vi "IOPanel_4.vi"(11 "IOCard In":refnum<class "IOCard.lvclass">) -> ()   [LabVIEW 2019]
uses:
  Ctrl/IO Card_Type.ctl
  IO_Class/IOCard.lvclass
  <vilib>/Utility/miscctls.llb/LVPositionTypeDef.ctl
  IO_Class/IOCard.lvclass/IOCard.ctl
  LLB/Message/Ctrl/MsgDataInput.ctl
  LLB/Message/Ctrl/MsgPageSelect.ctl
  LLB/Message/Ctrl/LogType.ctl
  IO_Class/6480/6480.lvclass
  C:/Users/MyUser/Desktop/204J1_20201007/System/Function/IO Folder/IO_Class/IOCard.lvclass
  IO_Class/2410C/2410C-64.lvclass
  IO_Class/Zan/ZanCard.lvclass
  IO_Class/DMC1000B/DMC1000B.lvclass
  IO_Class/16InOut/16InOut.lvclass
  global/InAndOutGB.vi
  LLB/Commonly VI/Main Glb.vi
  <vilib>/Utility/config.llb/Read Key (String).vi
  LLB/Commonly VI.lvlib
  <vilib>/Utility/config.llb/NI_LVConfig.lvlib
  LLB/Message/MsgShowAndLog.lvlib
panel:
  out "IOCard":refnum<class "IOCard.lvclass">
  out "Card_Type":T1
  out "QName":string
  in  "Tab Control":enum32{"Input", "Output"}(tab)
  out "Lst_Input":i32[](listbox) caption="Input"
  in  "Lst_Output":i32[](listbox)=[2] caption="Output"
  out "CardNumber":i32
  out "IOType":enum16{"Input", "Output"}(ring)=enum."Output"
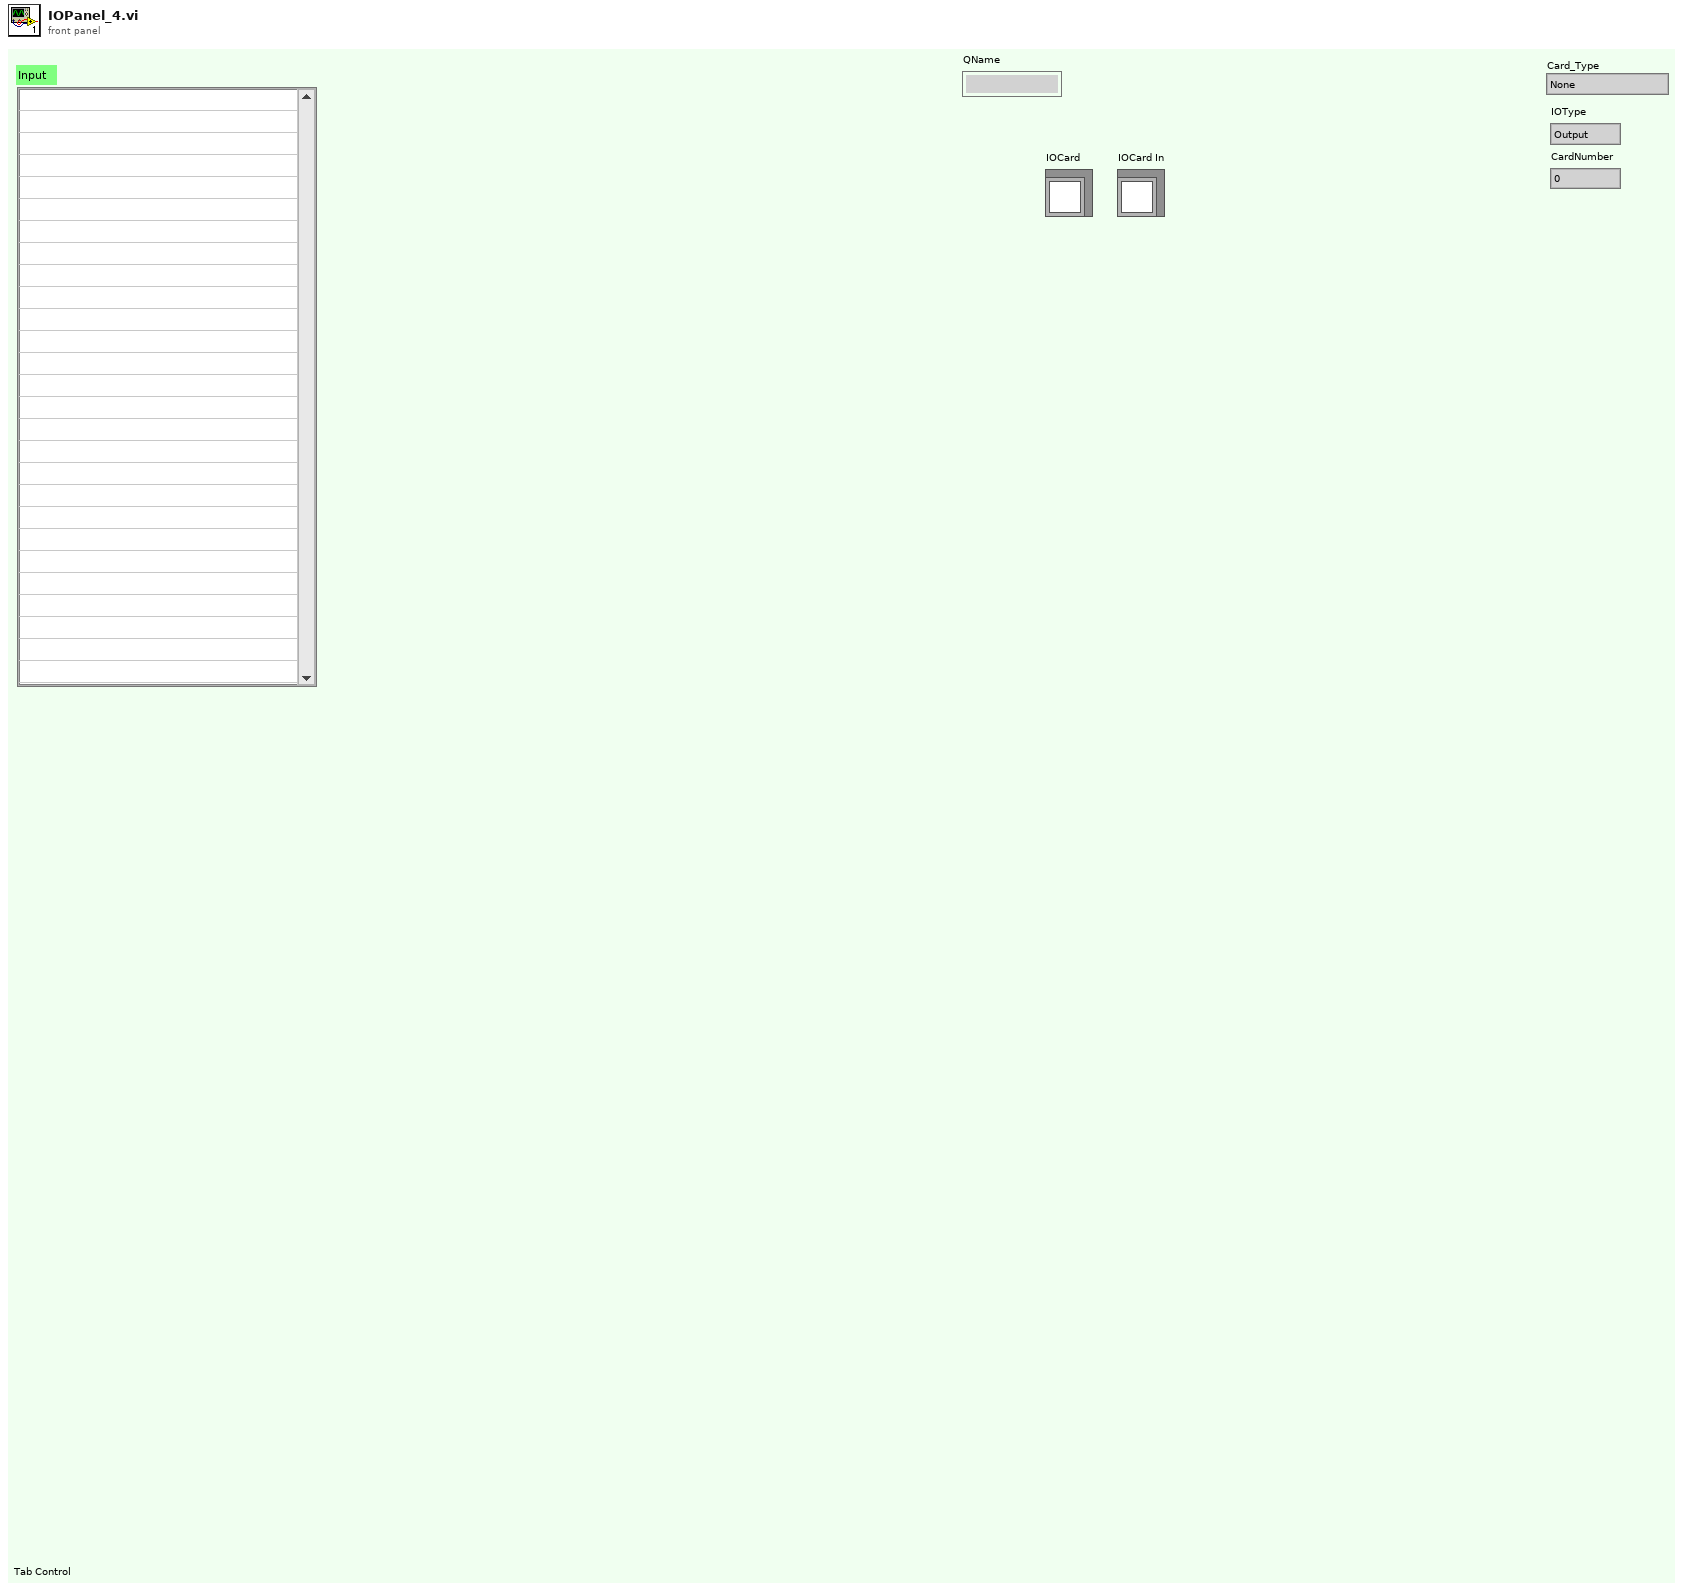
[diagram p1: front panel]
types:
  T1 = typedef "IO Card_Type.ctl" = enum16{"None", "Unidaq32", "6480", "2410C-64", "Zan", "DMC1000B", "16InOut", "Robot", "DMC3600"}
  T2 = typedef "LVPositionTypeDef.ctl" = cluster{"Left":i32, "Top":i32}
  T3 = cluster{"IO Card Type":T1, "IOType":enum16{"Input", "Output"}, "CardNumber":i32, "ConnectAct":bool, "IP":string}
  T4 = cluster{"CardNumber":i32, "Connect":bool, "Handler":i32}
  T5 = typedef "MsgDataInput.ctl" = cluster{"MsgPageSelect":T6, "LogType":T7, "Msg":string, "Time":string}
  T6 = typedef "MsgShowAndLog.lvlib/MsgPageSelect.ctl" = enum16{"System", "Comm", "IO", "Action", "Alarm"}
  T7 = typedef "MsgShowAndLog.lvlib/LogType.ctl" = enum16{"Auto", "Manual", "Handshake", "Error"}
  T8 = typedef "LVBoundsTypeDef.ctl" = cluster{"Width":u32, "Height":u32}
  T9 = typedef "LVPoint32TypeDef.ctl" = cluster{"Horizontal":i32, "Vertical":i32}
  T10 = typedef "NI_LVConfig.lvlib/Config Data RefNum.ctl" = refnum<k1>
  T11 = cluster{"Card":i32, "Connect":bool, "Handler":i32}[]
  T12 = cluster{"Card":i32, "Connect":bool, "Handler":i32}
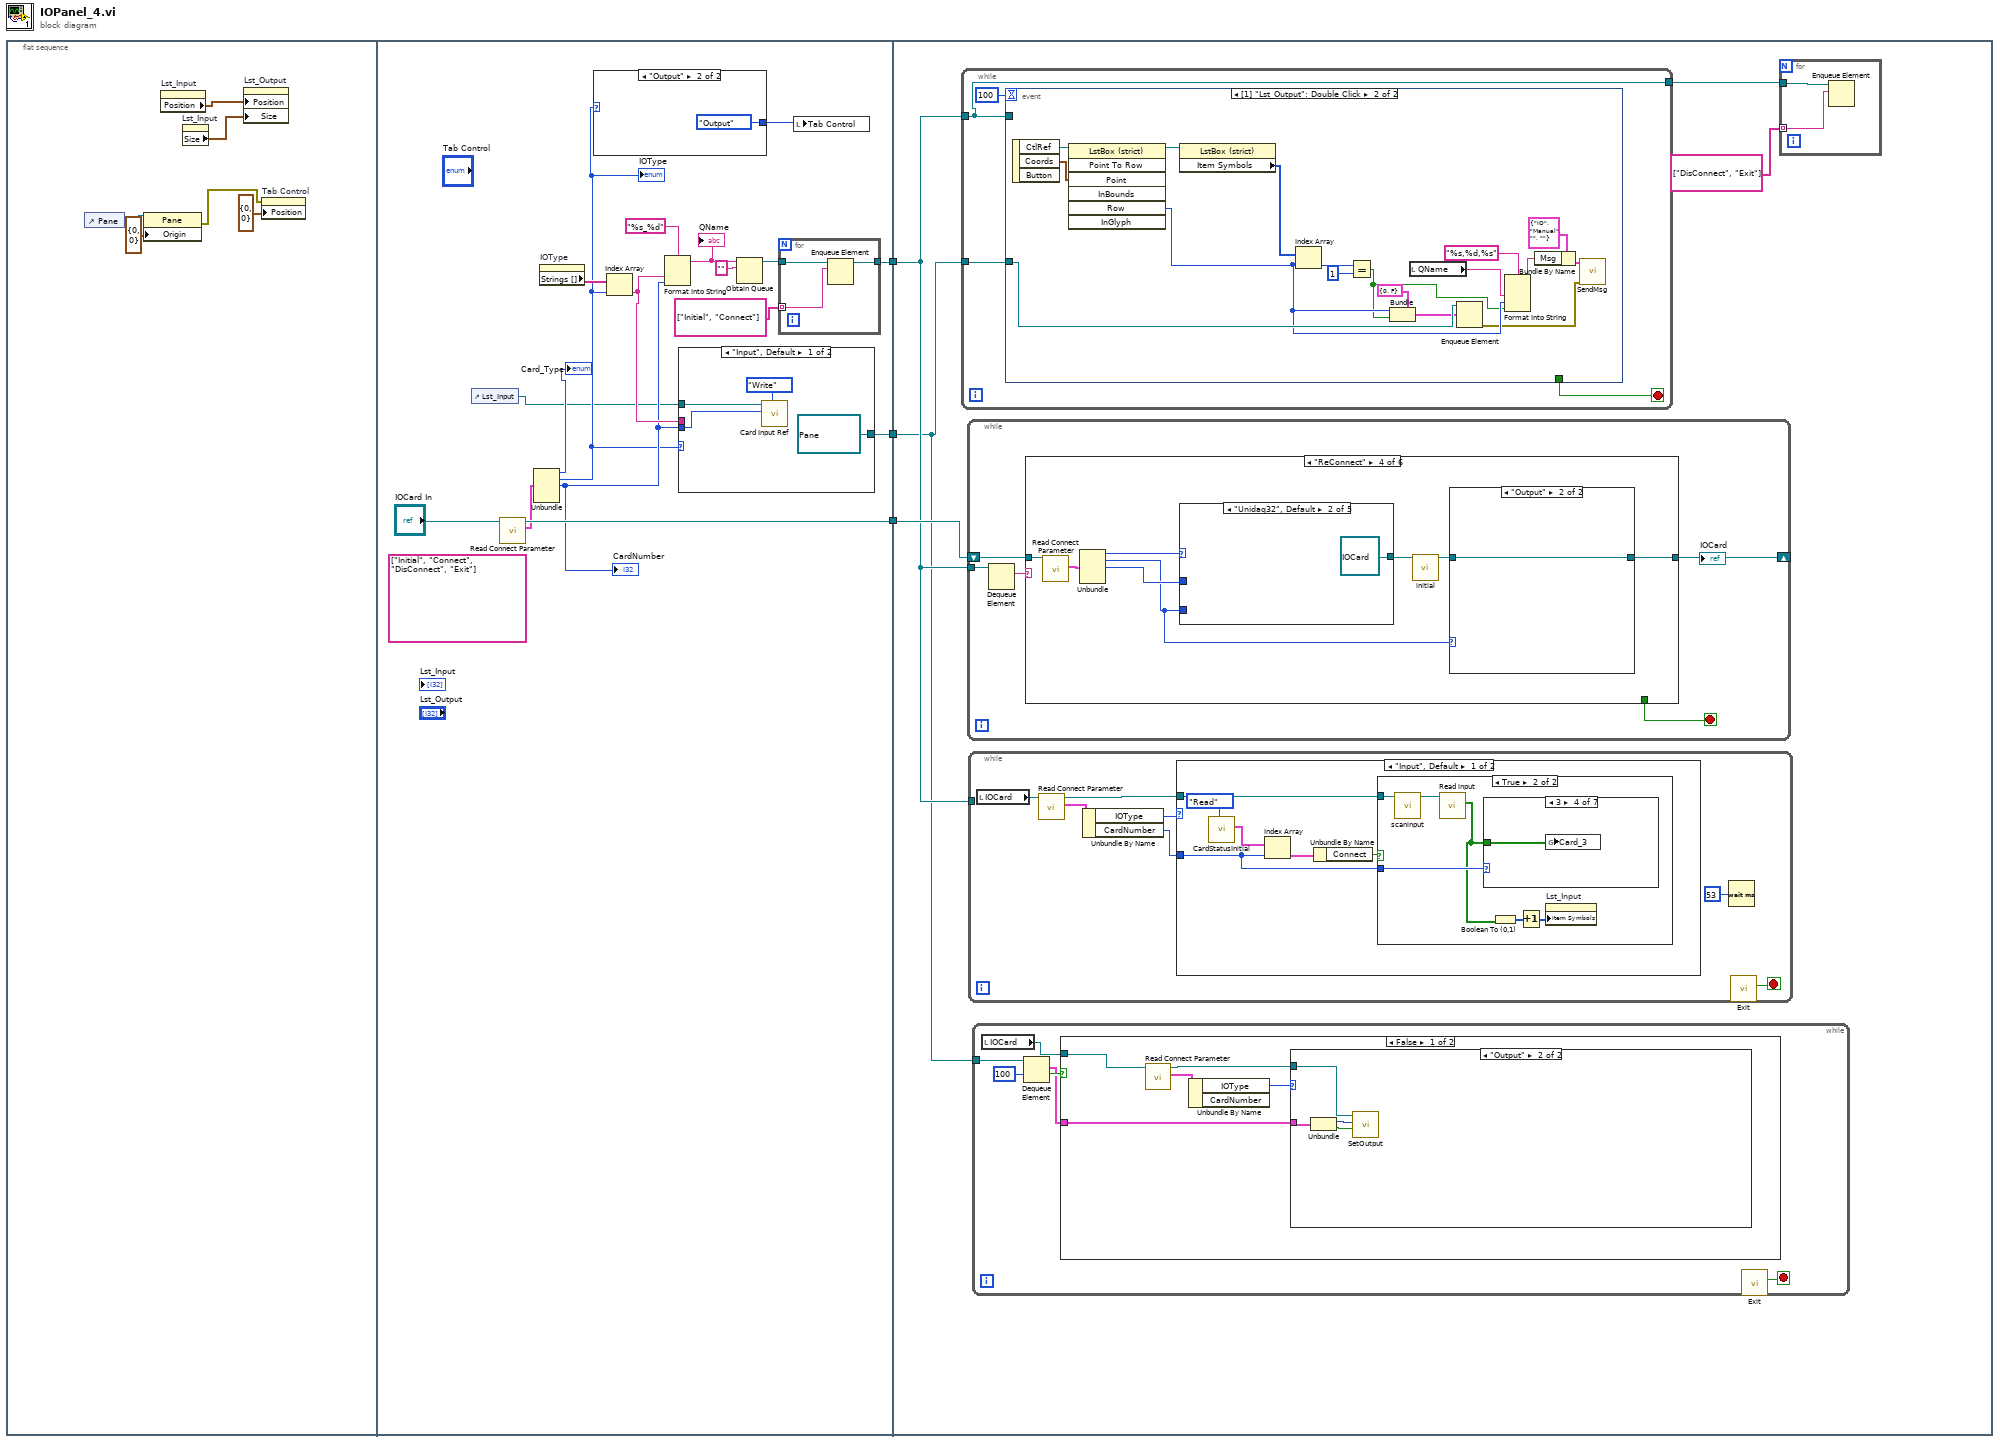
[diagram p0: block diagram]
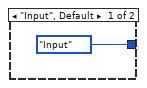
[diagram p2: hidden frame]
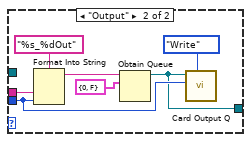
[diagram p3: hidden frame]
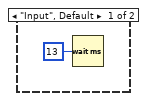
[diagram p4: hidden frame]
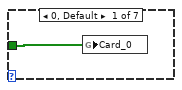
[diagram p7: hidden frame]
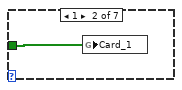
[diagram p8: hidden frame]
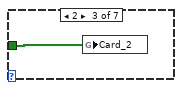
[diagram p9: hidden frame]
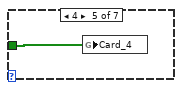
[diagram p10: hidden frame]
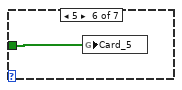
[diagram p11: hidden frame]
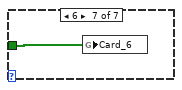
[diagram p12: hidden frame]
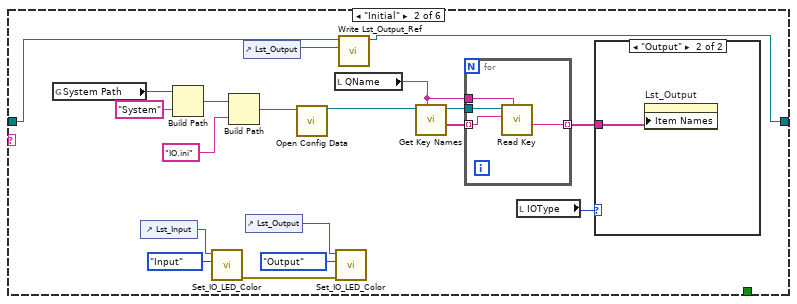
[diagram p15: hidden frame]
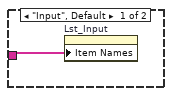
[diagram p16: hidden frame]
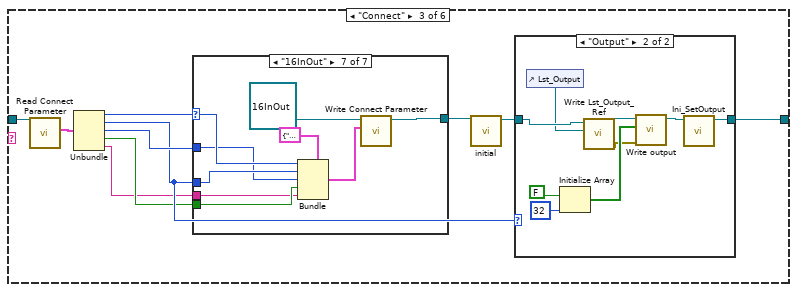
[diagram p17: hidden frame]
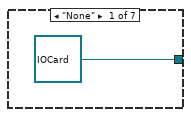
[diagram p19: hidden frame]
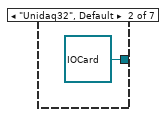
[diagram p20: hidden frame]
diagram:
  n1 = flat-sequence {
    tunnel: [w23] -> w3
    tunnel: [w18] -> w2
    tunnel: [w16] -> w1
    tunnel: w3 -> [w47]
    tunnel: w2 -> [w44]
    tunnel: w1 -> [w43]
    frame #0 {
      n2 = control-ref of="Pane"() -> (w6:refnum<vi>)
      n3 = property class="Pane"(reference=w6, "Origin"=T2 {"Left"=0, "Top"=0} ("Position")) -> (error out=w4:errorcluster)  [unwired: 1 in, 1 out]
      n4 = property on="Lst_Input" class="LstBox (strict)"() -> ("Position"=w8:T2)  [unwired: 2 in, 2 out]
      n5 = property on="Lst_Input" class="LstBox (strict)"() -> ("Size"=w9:T8)  [unwired: 2 in, 2 out]
      n6 = property on="Lst_Output" class="LstBox (strict)"("Position"=w8, "Size"=w9) -> ()  [unwired: 2 in, 2 out]
      n7 = property on="Tab Control" class="TabCtl (strict)"(error in=w4, "Position"=T2 {"Left"=0, "Top"=0}) -> ()  [unwired: 1 in, 2 out]
    }
    frame #1 {
      (unwired) string[] ["Initial", "Connect", "DisConnect", "Exit"]
      n8 = control-ref of="Lst_Input"() -> (w10:refnum<vi>)
      n9 = call "Read Connect Parameter.vi"("IOCard in"="IOCard In") -> ("Connect Parameter"=w22:T3, "IOCard out"=w23:refnum<class "IOCard.lvclass">)  [unwired: 8 in, 1 out]
      n10 = Unbundle(w22) -> ("IO Card Type"=→"Card_Type":T1, "IOType"=w12:enum16{"Input", "Output"}, "CardNumber"=w14:i32)  [unwired: 2 out]
      "CardNumber" <- w14
      "IOType" <- w12
      n11 = property on="IOType" class="Enum (strict)"() -> ("Strings []"=w21:string[])  [unwired: 2 in, 2 out]
      n12 = case shown="\"Output\"" w12 {
        tunnel: [enum32{"Input", "Output"}."Input" ("Tab Control") enum32{"Input", "Output"}."Output" ("Tab Control")] -> w11
        frame "Input", Default {
        }
        frame "Output" {
        }
      }
      n13 = Index Array(array=w21, index=w12) -> (element=w17:string)
      n14 = Format Into String(format string="%s_%d", w17, w14) -> (resulting string=w25:string)  [unwired: 2 in, 1 out]
      "QName" <- w25
      n15 = case shown="\"Input\", Default" w12 {
        tunnel: w17 -> [_ w37]
        tunnel: w14 -> [w29 w34]
        tunnel: [refnum<queue> refnum ("queue out") w33] -> w16
        tunnel: w10 -> [w30 _]
        frame "Input", Default {
          n16 = call "Card Input Ref.vi"("Action"=enum16{"Initial", "Write", "Read", "Release"}."Write", "CardIndex"=w29, "RefIn"=w30) -> ()  [unwired: 7 in, 2 out]
        }
        frame "Output" {
          n17 = Format Into String(format string="%s_%dOut", w37, w34) -> (resulting string=w39:string)  [unwired: 2 in, 1 out]
          n18 = Obtain Queue(name (unnamed)=w39, element data type=cluster{"Index":i32, "BL":bool} {"Index"=0, "BL"=FALSE}) -> (queue out=w33:refnum<queue>)  [unwired: 3 in, 2 out]
          n19 = call "Card Output Q.vi"("Action"=enum16{"Initial", "Write", "Read", "Release"}."Write", "CardIndex"=w34, "OutputQIn"=w33) -> ()  [unwired: 7 in, 2 out]
        }
      }
      n20 = Obtain Queue(name (unnamed)=w25, element data type="") -> (queue out=w19:refnum<queue>)  [unwired: 3 in, 2 out]
      n21 = for {
        tunnel: w19 -> [w42]
        tunnel: string[] ["Initial", "Connect"] -> [w41] mode=indexing
        tunnel: [w40] -> w18
        n22 = Enqueue Element(queue=w42, element=w41) -> (queue out=w40:refnum<queue>)  [unwired: 2 in, 2 out]
      }
      n23 = local write "Tab Control"(w11) -> ()
    }
    frame #2 {
      n24 = while {
        tunnel: w44 -> [w194]
        tunnel: [w194] -> w46
        tunnel: w43 -> [w193]
        stop <- w195 stop-if-true
        n25 = event shown="[1] \"Lst_Output\": Double Click" {
          selector: _ -> [_ _]
          dyn-events: _ -> [_ _]
          timeout: 100 -> [_ _]
          tunnel: [w197 _] -> w195
          tunnel: w194 -> [_ _]
          tunnel: w193 -> [_ w208]
          event Timeout {
            n26 = event-data() -> ()  [unwired: 1 in, 3 out]
            n27 = call "Exit.vi"() -> ("ExitOut"=w197:bool)  [unwired: 11 in]
          }
          event "Lst_Output": Double Click {
            n28 = event-data() -> ("CtlRef"=w214:refnum<vi>, "Coords"=w213:T9)  [unwired: 1 in, 1 out]
            n29 = invoke on="Invoke Node" class="LstBox (strict)" method="Point To Row"(reference=w214, "Point"=w213) -> (reference out=w209:refnum<vi>, "Row"=w200:i32)  [unwired: 5 in, 5 out]
            n30 = property on="Property Node" class="LstBox (strict)"(reference=w209) -> ("Item Symbols"=w212:i32[])  [unwired: 1 in, 2 out]
            n31 = Index Array(array=w212, index=w200) -> (element=w211:i32)
            n32 = Equal?(x=w211, y=1) -> (x = y?=w199:bool)
            n33 = Bundle(cluster=cluster{"Index":i32, "BL":bool} {"Index"=0, "BL"=FALSE} ("element"), "Index"=w200, "BL"=w199) -> (w207:cluster{"Index":i32, "BL":bool})
            n34 = local read "QName"() -> (w201:string)
            n35 = Enqueue Element(queue=w208, element=w207) -> (error out=w198:errorcluster)  [unwired: 2 in, 2 out]
            n36 = Format Into String(format string="%s,%d,%s", w201, w200, w199) -> (resulting string=w203:string)  [unwired: 2 in, 1 out]
            n37 = Bundle By Name(cluster=T5 {"MsgPageSelect"=enum."IO", "LogType"=enum."Manual", "Msg"="", "Time"=""} ("DataIn"), "Msg"=w203) -> (w205:T5)
            n38 = call "SendMsg.vi"("error in (no error)"=w198, "DataIn"=w205) -> ()  [unwired: 9 in, 1 out]
          }
        }
      }
      n39 = while {
        tunnel: w44 -> [w96]
        shift-right: [w94] -> _
        shift-left: w47 -> [w93]
        stop <- w92 stop-if-true
        n40 = Dequeue Element(queue=w96) -> (element=w95:string)  [unwired: 2 in, 3 out]
        n41 = case shown="\"ReConnect\"" w95 {
          tunnel: [w97 w99 w127 w168 w182 w191] -> w94
          tunnel: w93 -> [w97 w100 w132 w173 w183 w191]
          tunnel: [_ _ _ _ _ TRUE] -> w92
          frame "False", Default {
          }
          frame "Initial" {
            n42 = global read "Main Glb.vi" "System Path"() -> (w116:path)
            n43 = control-ref of="Lst_Input"() -> (w104:refnum<vi>)
            n44 = Build Path(base path=w116, name or relative path="System") -> (appended path=w114:path)
            n45 = call "Set_IO_LED_Color.vi"("SelectType"=enum16{"Input", "Output"}."Input", "ListBox Ref"=w104) -> ("error out"=w101:errorcluster)  [unwired: 9 in]
            n46 = Build Path(base path=w114, name or relative path="IO.ini") -> (appended path=w112:path)
            n47 = control-ref of="Lst_Output"() -> (w98:refnum<vi>)
            n48 = control-ref of="Lst_Output"() -> (w105:refnum<vi>)
            n49 = call <vilib>:"Open Config Data.vi"("configuration file path"=w112) -> ("refnum"=w111:T10)  [unwired: 8 in, 2 out]
            n50 = local read "QName"() -> (w108:string)
            n51 = call "Set_IO_LED_Color.vi"("error in (no error)"=w101, "SelectType"=enum16{"Input", "Output"}."Output", "ListBox Ref"=w105) -> ()  [unwired: 8 in, 1 out]
            n52 = call-dynamic "Write Lst_Output_Ref.vi"("Lst_Output_Ref"=w98, "IOCard in"=w100) -> ("IOCard out"=w99:refnum<class "IOCard.lvclass">)  [unwired: 8 in, 1 out]
            n53 = call <vilib>:"Get Key Names.vi"("section"=w108, "refnum"=w111) -> ("key names"=w109:string[], "refnum out"=w110:T10)  [unwired: 6 in, 2 out]
            n54 = for {
              tunnel: w110 -> [w122]
              tunnel: w109 -> [w121] mode=indexing
              tunnel: w108 -> [w120]
              tunnel: [w119] -> w106 mode=indexing
              n55 = call-poly <vilib>:"Read Key.vi"("section"=w120, "key"=w121, "refnum"=w122) -> ("value"=w119:string)  [unwired: 5 in, 3 out]
            }
            n56 = local read "IOType"() -> (w107:enum16{"Input", "Output"})
            n57 = case shown="\"Output\"" w107 {
              tunnel: w106 -> [w117 w118]
              frame "Input", Default {
                n58 = property on="Lst_Input" class="LstBox (strict)"("Item Names"=w117) -> ()  [unwired: 2 in, 2 out]
              }
              frame "Output" {
                n59 = property on="Lst_Output" class="LstBox (strict)"("Item Names"=w118) -> ()  [unwired: 2 in, 2 out]
              }
            }
          }
          frame "Connect" {
            n60 = call "Read Connect Parameter.vi"("IOCard in"=w132) -> ("Connect Parameter"=w131:T3)  [unwired: 8 in, 2 out]
            n61 = Unbundle(w131) -> ("IO Card Type"=w130:T1, "IOType"=w128:enum16{"Input", "Output"}, "CardNumber"=w129:i32, "ConnectAct"=w125:bool, "IP"=w124:string)
            n62 = case shown="\"16InOut\"" w130 {
              selector: w130 -> [_ _ _ _ _ w153 w162]
              tunnel: [refnum<class "IOCard.lvclass"> refnum ("IOCard.lvclass") refnum<class "IOCard.lvclass"> refnum ("IOCard.lvclass") refnum<class "6480.lvclass"> refnum ("6480.lvclass") refnum<class "2410C-64.lvclass"> refnum ("2410C-64.lvclass") refnum<class "ZanCard.lvclass"> refnum ("ZanCard.lvclass") w156 w165] -> w123
              tunnel: w129 -> [_ _ _ _ _ w151 w160]
              tunnel: w128 -> [_ _ _ _ _ w152 w161]
              tunnel: w125 -> [_ _ _ _ _ w150 w159]
              tunnel: w124 -> [_ _ _ _ _ w149 w158]
              frame "None" {
              }
              frame "Unidaq32", Default {
              }
              frame "6480" {
              }
              frame "2410C-64" {
              }
              frame "Zan" {
              }
              frame "DMC1000B" {
                w148 = refnum<class "DMC1000B.lvclass"> refnum  # DMC1000B.lvclass
                n63 = Bundle(cluster=T3 {"IO Card Type"=enum."None", "IOType"=enum."Output", "CardNumber"=0, "ConnectAct"=FALSE, "IP"=""} ("Connect Parameter"), "IO Card Type"=w153, "IOType"=w152, "CardNumber"=w151, "ConnectAct"=w150, "IP"=w149) -> (w154:T3)
                n64 = call "Write Connect Parameter.vi"("Connect Parameter"=w154, "IOCard in"=w148) -> ("IOCard out"=w156:refnum<class "DMC1000B.lvclass">)  [unwired: 8 in, 1 out]
              }
              frame "16InOut" {
                n65 = Bundle(cluster=T3 {"IO Card Type"=enum."None", "IOType"=enum."Output", "CardNumber"=0, "ConnectAct"=FALSE, "IP"=""} ("Connect Parameter"), "IO Card Type"=w162, "IOType"=w161, "CardNumber"=w160, "ConnectAct"=w159, "IP"=w158) -> (w163:T3)
                n66 = call "Write Connect Parameter.vi"("Connect Parameter"=w163, "IOCard in"=refnum<class "16InOut.lvclass"> refnum ("16InOut.lvclass")) -> ("IOCard out"=w165:refnum<class "16InOut.lvclass">)  [unwired: 8 in, 1 out]
              }
            }
            n67 = call-dynamic "initial.vi"("IOCard in"=w123) -> ("IOCard out"=w126:refnum<class "IOCard.lvclass">)  [unwired: 9 in, 1 out]
            n68 = case shown="\"Output\"" w128 {
              tunnel: [w133 w142] -> w127
              tunnel: w126 -> [w133 w136]
              frame "Input", Default {
              }
              frame "Output" {
                n69 = control-ref of="Lst_Output"() -> (w134:refnum<vi>)
                n70 = Initialize Array(FALSE, 32 ("dimension size")) -> (w140:bool[])
                n71 = call-dynamic "Write Lst_Output_Ref.vi"("Lst_Output_Ref"=w134, "IOCard in"=w136) -> ("error out"=w137:errorcluster, "IOCard out"=w135:refnum<class "IOCard.lvclass">)  [unwired: 8 in]
                n72 = call-dynamic "Write output.vi"("error in (no error)"=w137, "output"=w140, "IOCard in"=w135) -> ("IOCard out"=w141:refnum<class "IOCard.lvclass">)  [unwired: 7 in, 1 out]
                n73 = call-dynamic "Ini_SetOutput.vi"("IOCard in"=w141) -> ("IOCard out"=w142:refnum<class "IOCard.lvclass">)  [unwired: 9 in, 1 out]
              }
            }
          }
          frame "ReConnect" {
            n74 = call "Read Connect Parameter.vi"("IOCard in"=w173) -> ("Connect Parameter"=w172:T3)  [unwired: 8 in, 2 out]
            n75 = Unbundle(w172) -> ("IO Card Type"=w171:T1, "IOType"=w169:enum16{"Input", "Output"}, "CardNumber"=w170:i32)  [unwired: 2 out]
            n76 = case shown="\"Unidaq32\", Default" w171 {
              tunnel: [refnum<class "IOCard.lvclass"> refnum ("IOCard.lvclass") refnum<class "IOCard.lvclass"> refnum ("IOCard.lvclass") refnum<class "6480.lvclass"> refnum ("6480.lvclass") refnum<class "2410C-64.lvclass"> refnum ("2410C-64.lvclass") refnum<class "ZanCard.lvclass"> refnum ("ZanCard.lvclass")] -> w166
              tunnel: w170 -> [_ _ _ _ _]
              tunnel: w169 -> [_ _ _ _ _]
              frame "None" {
              }
              frame "Unidaq32", Default {
              }
              frame "6480" {
              }
              frame "2410C-64" {
              }
              frame "Zan" {
              }
            }
            n77 = call-dynamic "initial.vi"("IOCard in"=w166) -> ("IOCard out"=w167:refnum<class "IOCard.lvclass">)  [unwired: 9 in, 1 out]
            n78 = case shown="\"Output\"" w169 {
              tunnel: [w174 w175] -> w168
              tunnel: w167 -> [w174 w175]
              frame "Input", Default {
              }
              frame "Output" {
              }
            }
          }
          frame "DisConnect" {
            n79 = call "Read Connect Parameter.vi"("IOCard in"=w183) -> ("Connect Parameter"=w187:T3, "IOCard out"=w182:refnum<class "IOCard.lvclass">)  [unwired: 8 in, 1 out]
            n80 = Unbundle By Name(w187) -> ("CardNumber"=w184:i32, "IOType"=w181:enum16{"Input", "Output"})
            n81 = case shown="\"Output\"" w181 {
              tunnel: w183 -> [w189 _]
              frame "Input", Default {
                n82 = call-dynamic "close.vi"("IOCard in"=w189) -> ("error out"=w190:errorcluster)  [unwired: 9 in, 1 out]
                n83 = call <vilib>:"Clear Errors.vi"("error in (no error)"=w190) -> ()  [unwired: 5 in, 2 out]
              }
              frame "Output" {
              }
            }
            n84 = Bundle By Name(cluster=T4 {"CardNumber"=0, "Connect"=FALSE, "Handler"=0} ("DataIn"), "CardNumber"=w184) -> (w185:T4)
            n85 = call "CardStatusInitial.vi"("Action"=enum16{"Initial", "Write", "Read", "Release"}."Write", "DataIn"=w185, "CardNumber"=w184) -> ()  [unwired: 8 in, 1 out]
          }
          frame "Exit" {
          }
        }
        "IOCard" <- w94
      }
      n86 = while {
        tunnel: w44 -> [_]
        stop <- w69 stop-if-true
        n87 = local read "IOCard"() -> (w70:refnum<class "IOCard.lvclass">)
        n88 = call "Read Connect Parameter.vi"("IOCard in"=w70) -> ("Connect Parameter"=w67:T3, "IOCard out"=w68:refnum<class "IOCard.lvclass">)  [unwired: 8 in, 1 out]
        n89 = Unbundle By Name(w67) -> ("IOType"=w66:enum16{"Input", "Output"}, "CardNumber"=w65:i32)
        n90 = case shown="\"Input\", Default" w66 {
          tunnel: w68 -> [w76 _]
          tunnel: w65 -> [w71 _]
          frame "Input", Default {
            n91 = call "CardStatusInitial.vi"("Action"=enum16{"Initial", "Write", "Read", "Release"}."Read") -> ("CardStatus"=w74:T11)  [unwired: 10 in]
            n92 = Index Array(array=w74, index=w71) -> (element=w73:T12)
            n93 = Unbundle By Name(w73) -> ("Connect"=w72:bool)
            n94 = case shown="True" w72 {
              tunnel: w76 -> [_ w81]
              tunnel: w71 -> [_ w80]
              frame False {
              }
              frame True {
                n95 = call-dynamic "scaninput.vi"("IOCard in"=w81) -> ("IOCard out"=w82:refnum<class "IOCard.lvclass">)  [unwired: 9 in, 1 out]
                n96 = call-dynamic "Read input.vi"("IOCard in"=w82) -> ("input"=w79:bool[])  [unwired: 8 in, 2 out]
                n97 = case shown="3" w80 {
                  tunnel: w79 -> [w83 w84 w85 w86 w87 w88 w89]
                  frame 0, Default {
                    n98 = global write "InAndOutGB.vi" "Card_0"(w83) -> ()
                  }
                  frame 1 {
                    n99 = global write "InAndOutGB.vi" "Card_1"(w84) -> ()
                  }
                  frame 2 {
                    n100 = global write "InAndOutGB.vi" "Card_2"(w85) -> ()
                  }
                  frame 3 {
                    n101 = global write "InAndOutGB.vi" "Card_3"(w86) -> ()
                  }
                  frame 4 {
                    n102 = global write "InAndOutGB.vi" "Card_4"(w87) -> ()
                  }
                  frame 5 {
                    n103 = global write "InAndOutGB.vi" "Card_5"(w88) -> ()
                  }
                  frame 6 {
                    n104 = global write "InAndOutGB.vi" "Card_6"(w89) -> ()
                  }
                }
                n105 = Boolean To (0,1)(Boolean=w79) -> (0, 1=w78:i16[])
                n106 = Increment(x=w78) -> (x+1=w77:i16[])
                n107 = property on="Lst_Input" class="LstBox (strict)"("Item Symbols"=w77) -> ()  [unwired: 2 in, 2 out]
              }
            }
          }
          frame "Output" {
          }
        }
        n108 = Wait (ms)(milliseconds to wait=u32 53) -> ()  [unwired: 1 out]
        n109 = call "Exit.vi"() -> ("ExitOut"=w69:bool)  [unwired: 11 in]
      }
      n110 = while {
        tunnel: w43 -> [w52]
        stop <- w53 stop-if-true
        n111 = local read "IOCard"() -> (w48:refnum<class "IOCard.lvclass">)
        n112 = Dequeue Element(queue=w52, timeout in ms (-1)=100) -> (element=w49:cluster{"Index":i32, "BL":bool}, timed out?=w50:bool)  [unwired: 1 in, 2 out]
        n113 = case shown="False" w50 {
          tunnel: w49 -> [w55 _]
          tunnel: w48 -> [w54 _]
          frame False {
            n114 = call "Read Connect Parameter.vi"("IOCard in"=w54) -> ("Connect Parameter"=w58:T3, "IOCard out"=w56:refnum<class "IOCard.lvclass">)  [unwired: 8 in, 1 out]
            n115 = Unbundle By Name(w58) -> ("IOType"=w57:enum16{"Input", "Output"})  [unwired: 1 out]
            n116 = case shown="\"Output\"" w57 {
              tunnel: w56 -> [_ w62]
              tunnel: w55 -> [_ w63]
              frame "Input", Default {
                n117 = Wait (ms)(milliseconds to wait=u32 13) -> ()  [unwired: 1 out]
              }
              frame "Output" {
                n118 = Unbundle(w63) -> ("Index"=w61:i32, "BL"=w60:bool)
                n119 = call-dynamic "SetOutput.vi"("Boolean"=w60, "Index"=w61, "IOCard in"=w62) -> ()  [unwired: 6 in, 3 out]
              }
            }
          }
          frame True {
          }
        }
        n120 = call "Exit.vi"() -> ("ExitOut"=w53:bool)  [unwired: 11 in]
      }
      n121 = for {
        tunnel: w46 -> [w91]
        tunnel: string[] ["DisConnect", "Exit"] -> [w90] mode=indexing
        n122 = Enqueue Element(queue=w91, element=w90) -> ()  [unwired: 2 in, 3 out]
      }
    }
  }
